vi "Waveform Analysis (Events).vi"() -> ()   [LabVIEW 2012]
uses:
  <vilib>/Analysis/2dsp.llb/Real FFT.vi
  <vilib>/Analysis/NI_AALPro.lvlib
panel:
  out "Spectrum":dbl[](graph)
  out "Min":dbl
  out "Max":dbl
  out "Time Series":dbl[](graph)
  in  "Get Max & Min":bool
  in  "Calculate FFT":bool
  in  "Get Time Series":bool
  in  "Stop":bool
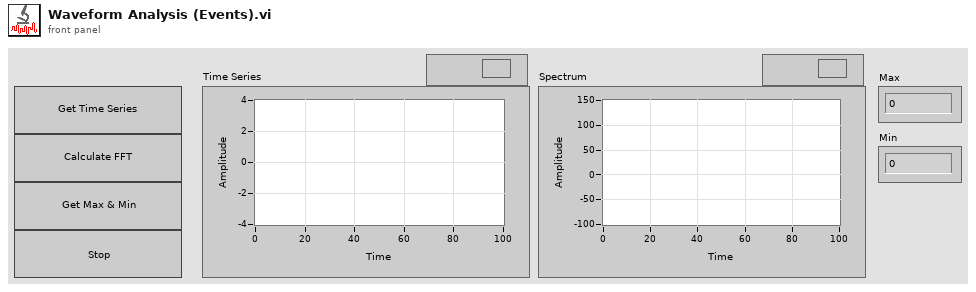
[diagram p1: front panel]
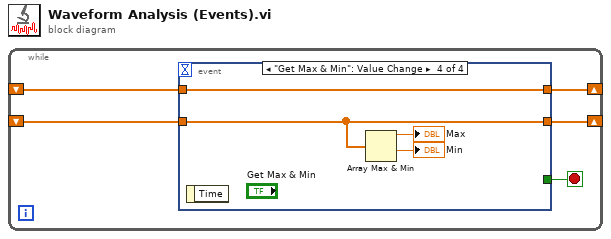
[diagram p0: block diagram]
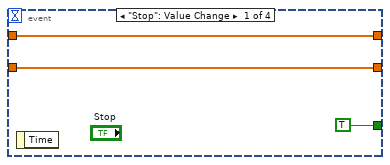
[diagram p2: hidden frame]
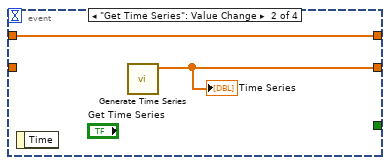
[diagram p3: hidden frame]
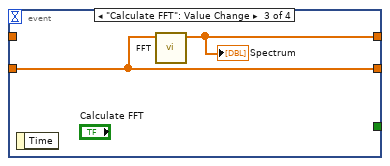
[diagram p4: hidden frame]
diagram:
  n1 = while {
    shift-right: [w4] -> _
    shift-left: _ -> [w3]
    shift-right: [w2] -> _
    shift-left: _ -> [w1]
    stop <- w5 stop-if-true
    n2 = event shown="[3] \"Get Max & Min\": Value Change" {
      selector: _ -> [_ _ _ _]
      dyn-events: _ -> [_ _ _ _]
      timeout: _ -> [_ _ _ _]
      tunnel: [TRUE _ _ _] -> w5
      tunnel: [w7 w9 w12 w15] -> w4
      tunnel: w3 -> [w7 _ w12 w15]
      tunnel: [w6 w10 w11 w16] -> w2
      tunnel: w1 -> [w6 w10 _ w16]
      event "Stop": Value Change {
        n3 = event-data() -> ()  [unwired: 1 in, 1 out]
      }
      event "Get Time Series": Value Change {
        n4 = event-data() -> ()  [unwired: 1 in, 1 out]
        n5 = call "Generate Time Series.vi"() -> ("Time Series"=w9:dbl[])  [unwired: 11 in]
        "Time Series" <- w9
      }
      event "Calculate FFT": Value Change {
        n6 = event-data() -> ()  [unwired: 1 in, 1 out]
        n7 = call-poly <vilib>:"FFT.vi"("X"=w12) -> ("FFT {X}"=w11:cdb[])  [unwired: 9 in, 1 out]
        "Spectrum" <- w11
      }
      event "Get Max & Min": Value Change {
        n8 = event-data() -> ()  [unwired: 1 in, 1 out]
        n9 = Array Max & Min(array=w15) -> (max value=→"Max":dbl, min value=→"Min":dbl)  [unwired: 2 out]
      }
    }
  }
